vi "shutdown.vi"(8 "error in (no error)":errorcluster, 11 "TCPCommunicator in":refnum<class "TCPCommunicator.lvclass">) -> (0 "error out":errorcluster, 3 "TCPCommunicator out":refnum<class "TCPCommunicator.lvclass">)   [LabVIEW 2016, in "TCPCommunicator.lvclass"]
uses:
  TCPCommunicator.lvclass
  TCPCommunicator.lvclass/TCPCommunicator.ctl
  TCPComEvents/TCPComEvents.lvclass
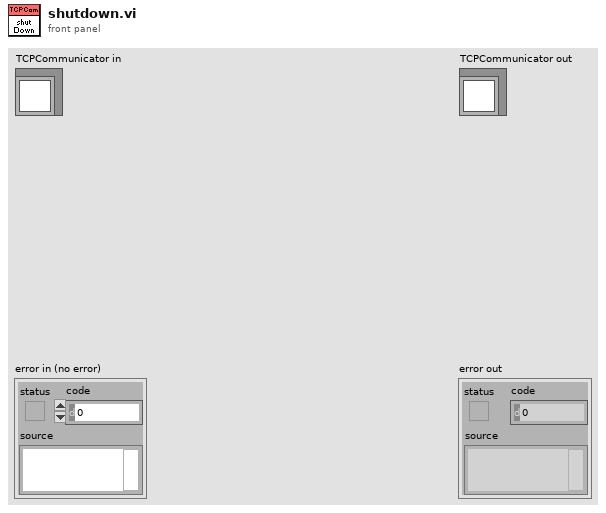
[diagram p1: front panel]
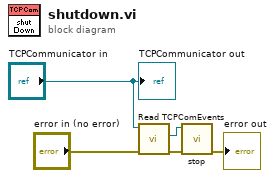
[diagram p0: block diagram]
diagram:
  n1 = call "Read TCPComEvents.vi"("error in (no error)"="error in (no error)", "TCPCommunicator in"="TCPCommunicator in") -> ("error out"=w3:errorcluster, "TCPComEvents.lvclass"=w4:refnum<class "TCPComEvents.lvclass">)  [unwired: 7 in, 1 out]
  n2 = call "stop.vi"("error in (no error)"=w3, "TCPComEvents in"=w4) -> ("error out"=→"error out":errorcluster)  [unwired: 8 in, 1 out]
  "TCPCommunicator out" <- "TCPCommunicator in"
